vi "Pulse Attribute, Log to Spreadsheet.vi"(5 "append to file (T)":bool=TRUE, 6 "error in":errorcluster, 8 "results file":path=path "C:/Documents and Settings/user/Desktop/Claytons Archive/results.txt", 9 "waveform file":path=path "C:/5-01-003 Active Electrode Min Max/Waveform 2 -0.02 mA") -> (0 "error out":errorcluster)   [LabVIEW 2010]
doc: "This function writes all of the waveform attributes to a spreadsheet file."
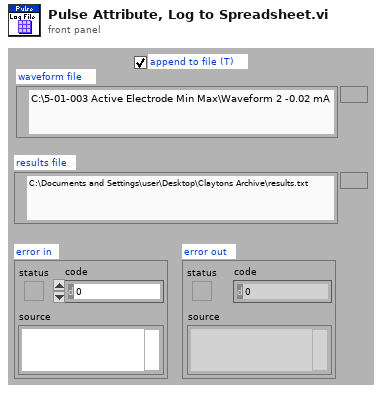
[diagram p1: front panel]
types:
  T1 = enum32{"existing file", "new file", "new or existing file", "existing dir", "new dir", "new or existing dir", "existing file (use LLBs)", "new file (use LLBs)", "new or existing file (use LLBs)", "new or existing file or directory (use LLBs)", "existing dir (use LLBs)", "new dir (use LLBs)", "new or existing dir (use LLBs)", "existing file or dir", "new file or dir", "new or existing file or dir", "existing file or dir (use LLBs)", "new file or dir (use LLBs)"}
  T2 = typedef "Waveform Attribute Cluster.ctl" = cluster{"Label":string, "Value":dbl}
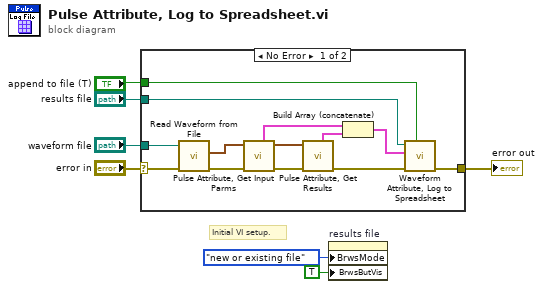
[diagram p0: block diagram]
diagram:
  # "Initial VI setup."
  n1 = case shown="No Error" "error in" {
    selector: "error in" -> [w20 w21]
    tunnel: [w11 w21] -> w7
    tunnel: "waveform file" -> [w18 _]
    tunnel: "results file" -> [w10 _]
    tunnel: "append to file (T)" -> [w9 _]
    frame No Error {
      n2 = call <vilib>:"Read Waveform from File.vi"("error in (no error)"=w20, "file path (dialog if empty)"=w18) -> ("error out"=w19:errorcluster, "first waveform in record"=w8:waveform(dbl))  [unwired: 4 in, 2 out]
      n3 = call "Pulse Attribute, Get Input Parms.vi"("error in"=w19, "waveform"=w8) -> ("error out"=w17:errorcluster, "waveform dup"=w16:waveform(dbl), "input parameters"=w14:T2[])  [unwired: 5 in]
      n4 = call "Pulse Attribute, Get Results.vi"("error in"=w17, "waveform"=w16) -> ("error out"=w12:errorcluster, "Results"=w15:T2[])  [unwired: 5 in, 1 out]
      n5 = Build Array (concatenate)(w14, w15) -> (w13:T2[])
      n6 = call "Waveform Attribute, Log to Spreadsheet.vi"("append to file (T)"=w9, "error in"=w12, "attributes"=w13, "results file"=w10) -> ("error out"=w11:errorcluster)  [unwired: 3 in, 2 out]
    }
    frame Error {
    }
  }
  "error out" <- w7
  n7 = property on="results file" class="Path"("BrwsMode"=T1."new or existing file" ("Browse Options:Selection Mode"), "BrwsButVis"=TRUE ("Browse Button:Visible")) -> ()  [unwired: 2 in, 2 out]
